vi "RT Main.vi"() -> ()   [LabVIEW 2025]
uses:
  FPGA IP/Types/PWM.Measure.Digital.Result.ctl
  FPGA IP/Types/PWM.Generate.Digital.Convert.Settings.ctl
  <vilib>/Platform/TimedLoop/XDataNode/timing_clust.ctl
  <vilib>/Platform/TimedLoop/XDataNode/nitl_modes.ctl
  <vilib>/Platform/TimedLoop/XDataNode/wakeup.ctl
  <vilib>/DAQmx/read.llb/DAQmx Read (Analog 1D Wfm NChan NSamp).vi
  <vilib>/Platform/TimedLoop/XDataNode/loadnilvce.vi
  <vilib>/FPGAPlugInAG/cRIO-9045/niLvFpga_Open_cRIO-9045.vi
  <vilib>/rvi/interface/common/dynamic/niFpgaDynamicAddResources.vi
  <vilib>/DAQmx/create/channels.llb/DAQmx Create Channel (AI-Voltage-Basic).vi
  <vilib>/DAQmx/configure/timing.llb/DAQmx Timing (Sample Clock).vi
  <vilib>/DAQmx/miscellaneous.llb/DAQmx Fill In Error Info.vi
  <vilib>/Utility/error.llb/Error Cluster From Error Code.vi
  <vilib>/rvi/errors/niLvFpgaAdjustHostInterfaceError.vi
  <vilib>/FPGAPlugInAG/Dynamic/niLvFpga_Close_Dynamic.vi
  <vilib>/platform/TimedLoop/XDataNode/XDataNode.xnode
  <vilib>/rvi/interface/nirviOpenFPGA/nirviOpenFPGA.xnode
  FPGA Bitfiles/finalapplication_FPGATarget_FPGAMain_-poiTnE8a14.lvbitx
  <vilib>/rvi/interface/nirviReadWriteControl/nirviReadWriteControl.xnode
  <vilib>/rvi/interface/nirviCloseFPGA/nirviCloseFPGA.xnode
  <resource>/objmgr/daqmx.rc
  <vilib>/Platform/TimedLoop/XDataNode/XDNodeRunTimeDep.lvlib
  <vilib>/rvi/interface/Simulation/niFpgaSimulationCallBeginRW.vi
  FPGA IP/Speciality FPGA IO.lvlib
  NiFpgaLv.dll
panel:
  out "error out":errorcluster
  in  "Mod2 DI0 PWM AcqSettings":cluster{"ACTIVE EDGE":bool, "TIMEOUT":u32}={"ACTIVE EDGE"=TRUE, "TIMEOUT"=40000000}
  in  "Mod2 DI3 PWM AcqSettings":cluster{"ACTIVE EDGE":bool, "TIMEOUT":u32}={"ACTIVE EDGE"=TRUE, "TIMEOUT"=40000000}
  in  "stop PWM":bool
  in  "Mod1 PWM Gen Settings":T1={"ACTIVE EDGE"=TRUE, "FREQ"=500.0, "DC"=50.0}
  in  "Mod2 PWM Gen Settings":T1={"ACTIVE EDGE"=TRUE, "FREQ"=10000.0, "DC"=25.0}
  out "Mod2 DI0 PWM Measurement":T2
  out "Mod2 DI3 PWM Measurement":T2
  in  "stop control":bool
  out "AI0":dbl
  in  "AO0":dbl
  in  "stop acq":bool
  out "Acquired Data Graph":waveform(dbl)[](graph)
  out "Actual AI Sample Rate":dbl
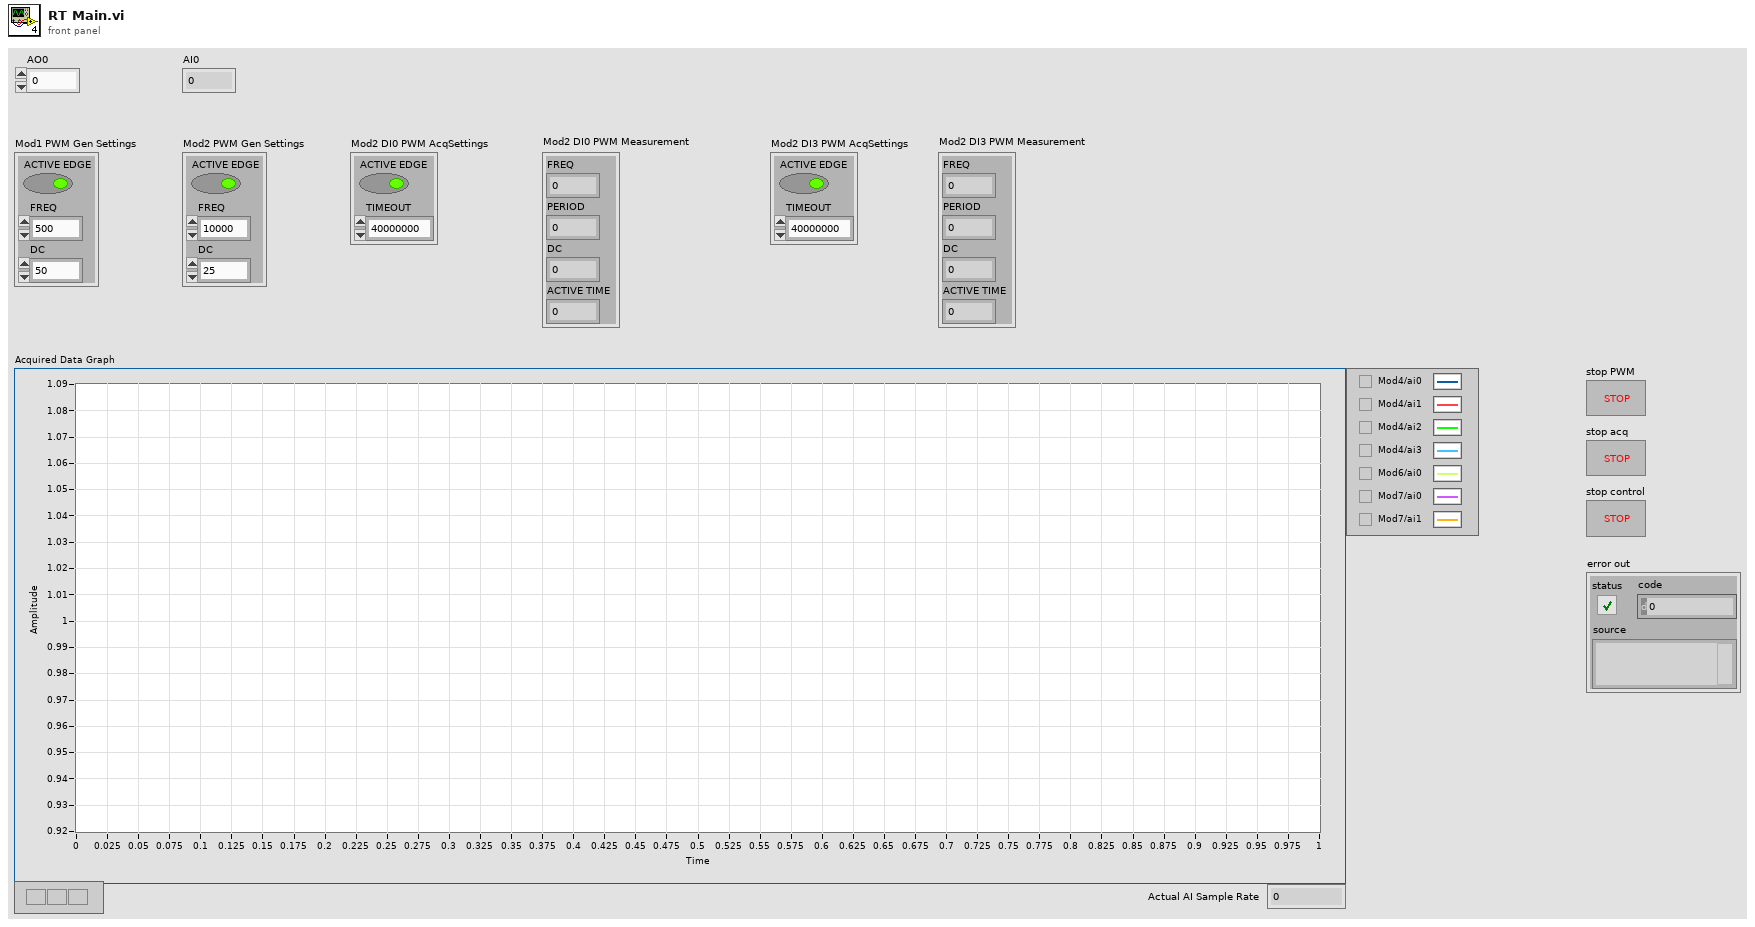
[diagram p1: front panel]
types:
  T1 = typedef "Speciality FPGA IO.lvlib/PWM.Generate.Digital.Convert.Settings.ctl" = cluster{"ACTIVE EDGE":bool, "FREQ":sgl, "DC":sgl}
  T2 = typedef "Speciality FPGA IO.lvlib/PWM.Measure.Digital.Result.ctl" = cluster{"FREQ":sgl, "PERIOD":sgl, "DC":sgl, "ACTIVE TIME":sgl}
  T3 = typedef "Speciality FPGA IO.lvlib/PWM.Generate.Digital.Settings.ctl" = cluster{"ACTIVE EDGE":bool, "ACTIVE TICKS":u32, "INACTIVE TICKS":u32}
  T4 = cluster{"ACTIVE TICKS":u32, "INACTIVE TICKS":u32, "ACQ TICKS":u32}
  T5 = typedef "XDNodeRunTimeDep.lvlib/timing_clust.ctl" = cluster{"Expected End [f-1]":u64, "Actual End [f-1]":u64, "Finished Late? [f-1]":bool, "Expected End [i-1]":u64, "Actual End [i-1]":u64, "Finished Late? [i-1]":bool, "Expected Start [i]":u64, "Actual Start [i]":u64, "Expected Start [f]":u64, "Actual Start [f]":u64, "Source Name":string, "Structure Name":string, "Period":i64, "Deadline":i64, "Offset":i64, "Start":i64, "Priority":i32, "Timeout":i32, "Mode":T6, "Wakeup Reason":T7, "Error":errorcluster, "Source Type":string, "Secondary Source Type":string, "Global End Time":u64, "Global Start Time":u64, "Frame Duration":u64, "Iteration Duration":u64, "Assigned CPU":i32, "I/O Scan Engine Mode":u32}
  T6 = typedef "XDNodeRunTimeDep.lvlib/nitl_modes.ctl" = enum32{"No Change", "Process missed periods, maintain original phase", "Discard missed periods, maintain original phase", "Process missed periods, ignore original phase", "Discard missed periods, ignore original phase"}
  T7 = typedef "XDNodeRunTimeDep.lvlib/wakeup.ctl" = enum32{"Normal", "Aborted", "Asynchronous wakeup", "Timing source error", "Timed loop error", "Timeout"}
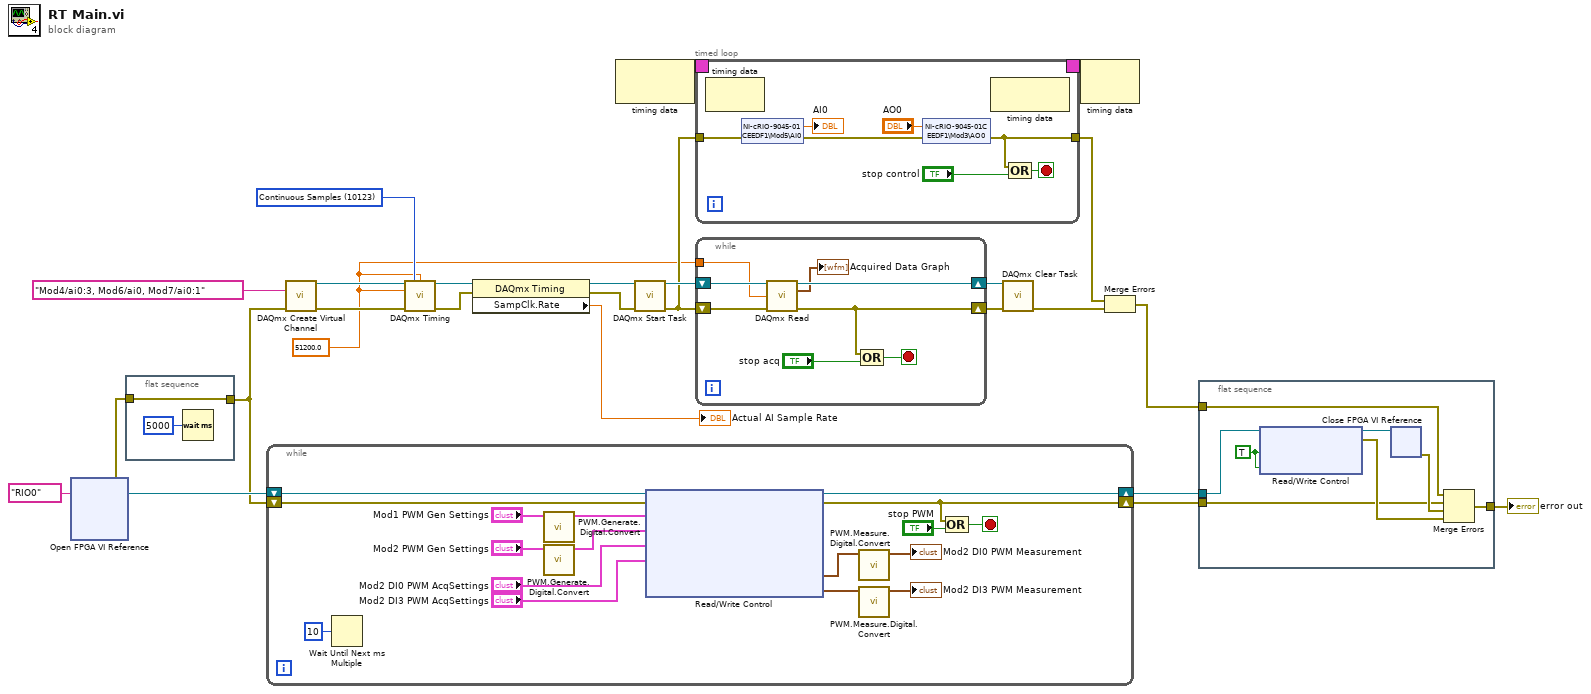
[diagram p0: block diagram]
diagram:
  w1 = 51200.0 ("rate")
  w23 = 10123 items=["Finite Samples"=10178, "Continuous Samples"=10123, "Hardware Timed Single Point"=12522] ("sample mode")
  n1 = xnode "Open FPGA VI Reference"("resource name"=tag "RIO0") -> ("FPGA VI Reference Out"=w10:refnum<k20>, "error out"=w3:errorcluster)  [unwired: 1 in]
  n2 = flat-sequence {
    tunnel: w3 -> [w27]
    tunnel: [w27] -> w2
    frame #0 {
      n3 = Wait (ms)(milliseconds to wait=u32 5000) -> ()  [unwired: 1 out]
    }
  }
  n4 = while {
    shift-right: [w43] -> w9
    shift-left: w10 -> [w45]
    shift-right: [w39] -> w8
    shift-left: w2 -> [w44]
    stop <- w37 stop-if-true
    n5 = Wait Until Next ms Multiple(millisecond multiple=u32 10) -> ()  [unwired: 1 out]
    n6 = call "PWM.Generate.Digital.Convert.vi"("Settings"="Mod1 PWM Gen Settings") -> ("Settings"=w36:T3)  [unwired: 10 in]
    n7 = call "PWM.Generate.Digital.Convert.vi"("Settings"="Mod2 PWM Gen Settings") -> ("Settings"=w34:T3)  [unwired: 10 in]
    n8 = xnode "Read/Write Control"("FPGA VI Reference In"=w45, "error in"=w44, "Mod1 PWM Gen Settings"=w36, "Mod2 PWM Gen Settings"=w34, "Mod2 DI0 PWM AcqSettings"="Mod2 DI0 PWM AcqSettings", "Mod2 DI3 PWM AcqSettings"="Mod2 DI3 PWM AcqSettings") -> ("FPGA VI Reference Out"=w43:refnum<k20>, "error out"=w39:errorcluster, "Mod2 DI0 PWM Measurement"=w32:T4, "Mod2 DI3 PWM Measurement"=w31:T4)
    n9 = call "PWM.Measure.Digital.Convert.vi"("Measurement"=w32) -> ("Result"=→"Mod2 DI0 PWM Measurement":T2)  [unwired: 10 in]
    n10 = call "PWM.Measure.Digital.Convert.vi"("Measurement"=w31) -> ("Result"=→"Mod2 DI3 PWM Measurement":T2)  [unwired: 10 in]
    n11 = Compound Arithmetic op=OR(w39, "stop PWM") -> (w37:bool)
  }
  n12 = call-poly <vilib>:"DAQmx Create Virtual Channel.vi"("physical channels"=tag "Mod4/ai0:3, Mod6/ai0, Mod7/ai0:1", "error in"=w2) -> ("task out"=w25:refnum<k21>, "error out"=w24:errorcluster)  [unwired: 12 in]
  n13 = call-poly <vilib>:"DAQmx Timing.vi"("task/channels in"=w25, "sample mode"=w23, "samples per channel"=w1, "rate"=w1, "error in"=w24) -> ("task out"=w22:refnum<k21>, "error out"=w18:errorcluster)  [unwired: 9 in]
  n14 = property class="DAQmx Timing"(reference=w22, error in=w18) -> (reference out=w16:refnum<k21>, error out=w15:errorcluster, "SampClk.Rate"=→"Actual AI Sample Rate":dbl)
  n15 = node-c288() -> (w14:T5)  [unwired: 1 in]
  n16 = call <vilib>:"DAQmx Start Task.vi"("task/channels in"=w16, "error in"=w15) -> ("task out"=w21:refnum<k21>, "error out"=w12:errorcluster)  [unwired: 12 in]
  n17 = timed-loop {
    timing: w14 -> [_]
    timing-out: [_] -> w13
    tunnel: w12 -> [w49]
    tunnel: [w46] -> w6
    stop <- w47 stop-if-true
    n18 = node-c288() -> ()  [unwired: 1 in, 1 out]
    n19 = shared-variable "NI-cRIO-9045-01CEEDF1\\Mod5\\AI0"(error in=w49) -> (→"AI0":dbl, error out=w51:errorcluster)
    n20 = shared-variable "NI-cRIO-9045-01CEEDF1\\Mod3\\AO0"("AO0", error in=w51) -> (error out=w46:errorcluster)
    n21 = node-c288() -> ()  [unwired: 1 in, 1 out]
    n22 = Compound Arithmetic op=OR(w46, "stop control") -> (w47:bool)
  }
  n23 = while {
    shift-right: [w60] -> w20
    shift-left: w21 -> [w62]
    shift-right: [w58] -> w19
    shift-left: w12 -> [w61]
    tunnel: w1 -> [w55]
    stop <- w56 stop-if-true
    n24 = call-poly <vilib>:"DAQmx Read.vi"("task/channels in"=w62, "number of samples per channel"=w55, "error in"=w61) -> ("task out"=w60:refnum<k21>, "data"=→"Acquired Data Graph":waveform(dbl)[], "error out"=w58:errorcluster)  [unwired: 10 in]
    n25 = Compound Arithmetic op=OR(w58, "stop acq") -> (w56:bool)
  }
  n26 = call <vilib>:"DAQmx Clear Task.vi"("task in"=w20, "error in"=w19) -> ("error out"=w5:errorcluster)  [unwired: 13 in]
  n27 = node-c288(w13) -> ()  [unwired: 1 out]
  n28 = Merge Errors(w6, w5) -> (w4:errorcluster)
  n29 = flat-sequence {
    tunnel: w9 -> [w70]
    tunnel: w8 -> [w65]
    tunnel: [w64] -> w7
    tunnel: w4 -> [w63]
    frame #0 {
      w69 = TRUE ("Stop Slow PWM")
      n30 = xnode "Read/Write Control"("FPGA VI Reference In"=w70, "Stop Slow PWM"=w69, "Stop Fast PWM"=w69) -> ("FPGA VI Reference Out"=w68:refnum<k20>, "error out"=w66:errorcluster)  [unwired: 1 in]
      n31 = xnode "Close FPGA VI Reference"("FPGA VI Reference In"=w68) -> ("error out"=w67:errorcluster)  [unwired: 1 in]
      n32 = Merge Errors(w63, w65, w67, w66) -> (w64:errorcluster)
    }
  }
  "error out" <- w7
